vi "Position_Globals.vi"() -> ()   [LabVIEW 2018]
panel:
  out "Zero_Position":bool
  in  "Robot_Y":dbl
  in  "Robot_X":dbl
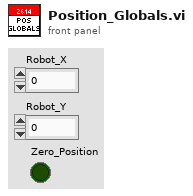
[diagram p1: front panel]
diagram:
